vi "PropagateOffset.vi"(10 "AmplifierSim.lvclass":refnum<class "AmplifierSim.lvclass">, 11 "MultimeterSim.lvclass":refnum<class "MultimeterSim.lvclass">) -> (3 "MultimeterSimOut":refnum<class "MultimeterSim.lvclass">)   [LabVIEW 2017, in "MultimeterSim.lvclass"]
uses:
  MultimeterSim.lvclass
  AmplifierSim.lvclass
  MultimeterSim.lvclass/MultimeterSim.ctl
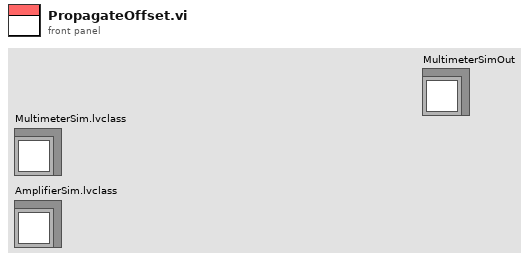
[diagram p1: front panel]
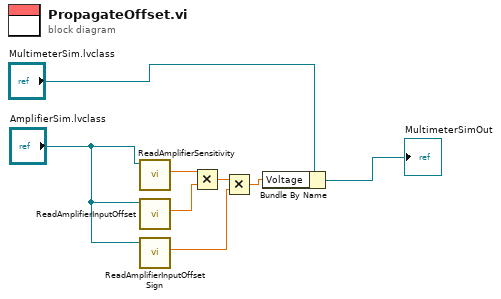
[diagram p0: block diagram]
diagram:
  n1 = call-dynamic "ReadAmplifierSensitivity.vi"("AmplifierSim in"="AmplifierSim.lvclass") -> ("Sensitivity"=w7:dbl)  [unwired: 8 in, 2 out]
  n2 = call-dynamic "ReadAmplifierInputOffset.vi"("AmplifierSim in"="AmplifierSim.lvclass") -> ("Input Offset"=w6:dbl)  [unwired: 8 in, 2 out]
  n3 = call-dynamic "ReadAmplifierInputOffsetSign.vi"("AmplifierSim in"="AmplifierSim.lvclass") -> ("Input Offset Sign"=w4:dbl)  [unwired: 8 in, 2 out]
  n4 = Multiply(x=w7, y=w6) -> (x*y=w5:dbl)
  n5 = Multiply(x=w5, y=w4) -> (x*y=w2:dbl)
  n6 = Bundle By Name(cluster="MultimeterSim.lvclass", "Voltage"=w2) -> (→"MultimeterSimOut":refnum<class "MultimeterSim.lvclass">)
